vi "Execute (Tree).vi"(8 "error in (no error)":errorcluster, 9 "Tree in":refnum<class "Tree.lvclass">, 10 "Expression":string, 11 "Data in":refnum<class "Data.lvclass">) -> (0 "error out":errorcluster, 1 "Tree out":refnum<class "Tree.lvclass">, 2 "Returned data out":refnum<class "Data.lvclass">, 3 "Data out":refnum<class "Data.lvclass">)   [LabVIEW 2012, in "MDSplus.lvlib" / "Data.lvclass"]
doc: "Compile and evaluate expression."
uses:
  <vilib>/MDSplus/Classes/Data_Class/Data.lvclass
  <vilib>/MDSplus/Classes/Tree_Class/Tree.lvclass
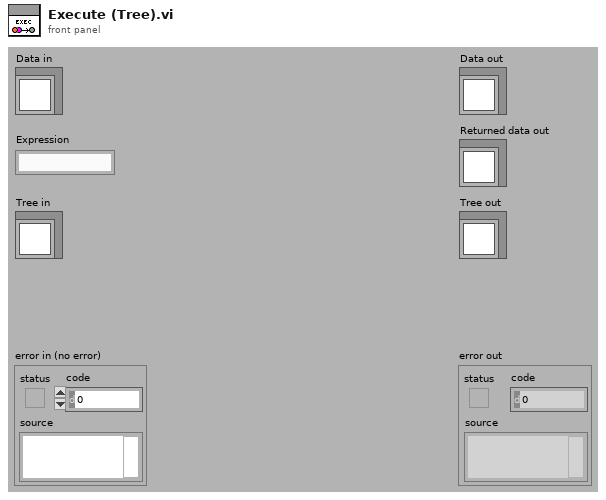
[diagram p1: front panel]
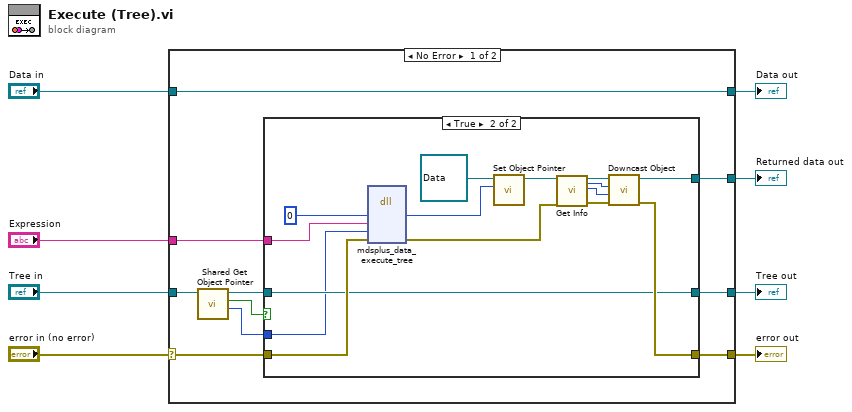
[diagram p0: block diagram]
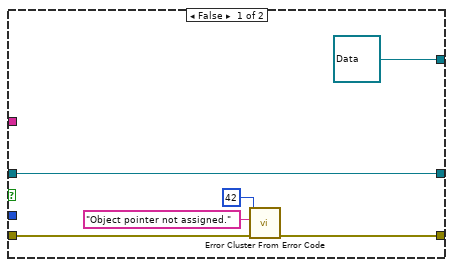
[diagram p2: hidden frame]
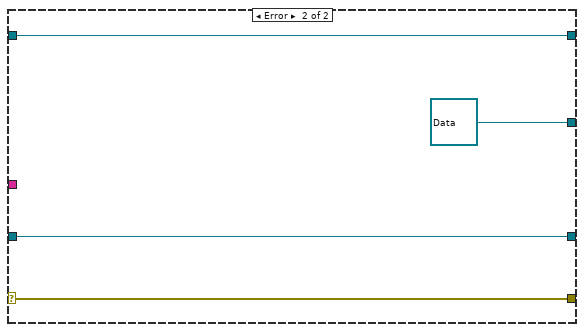
[diagram p3: hidden frame]
diagram:
  n1 = case shown="No Error" "error in (no error)" {
    selector: "error in (no error)" -> [w17 w43]
    tunnel: [w16 w43] -> w7
    tunnel: "Expression" -> [w18 _]
    tunnel: [w15 refnum<class "Data.lvclass"> refnum ("MDSplus.lvlib:Data.lvclass")] -> w5
    tunnel: "Tree in" -> [w14 w41]
    tunnel: [w11 w41] -> w4
    tunnel: [w9 w40] -> w2
    tunnel: "Data in" -> [w9 w40]
    frame No Error {
      n2 = call <vilib>:"Shared Get Object Pointer.vi"("Tree in"=w14) -> ("Object Pointer"=w10:i64, "Assigned object pointer?"=w13:bool, "Tree out"=w12:refnum<class "Tree.lvclass">)  [unwired: 8 in]
      n3 = case shown="True" w13 {
        tunnel: w18 -> [_ w39]
        tunnel: w17 -> [w21 w38]
        tunnel: [w20 w28] -> w16
        tunnel: [refnum<class "Data.lvclass"> refnum ("Data out") w27] -> w15
        tunnel: w12 -> [w24 w26]
        tunnel: [w24 w26] -> w11
        tunnel: w10 -> [_ w25]
        frame False {
          n4 = call <vilib>:"Error Cluster From Error Code.vi"("error in (no error)"=w21, "error message (\"\")"="Object pointer not assigned." ("error message (\"\")"), "error code (0)"=42) -> ("error out"=w20:errorcluster)  [unwired: 6 in]
        }
        frame True {
          n5 = dll-call lib="MDSobjectsLVShr" fn="mdsplus_data_execute_tree"("lvDataPtrOut"=i64 0 ("lvTreeNodePtr"), "exprIn"=w39, "lvTreePtrIn"=w25, "error"=w38) -> ("lvDataPtrOut"=w30:i64, "error"=w29:errorcluster)  [unwired: 6 in, 2 out]
          n6 = call-dynamic "Set Object Pointer.vi"("Object Pointer"=w30, "Data in"=refnum<class "Data.lvclass"> refnum ("Data.lvclass")) -> ("Data out"=w35:refnum<class "Data.lvclass">)  [unwired: 9 in]
          n7 = call-dynamic "Get Info.vi"("Data in"=w35, "error in (no error)"=w29) -> ("Data out"=w34:refnum<class "Data.lvclass">, "Class type out"=w33:u8, "Data type out"=w32:u8, "error out"=w31:errorcluster)  [unwired: 12 in, 2 out]
          n8 = call <vilib>:"Downcast Object.vi"("error in (no error)"=w31, "Data Type"=w32, "Class Type"=w33, "Data in"=w34) -> ("error out"=w28:errorcluster, "Data out"=w27:refnum<class "Data.lvclass">)  [unwired: 6 in]
        }
      }
    }
    frame Error {
    }
  }
  "error out" <- w7
  "Returned data out" <- w5
  "Tree out" <- w4
  "Data out" <- w2
